vi "Filling.vi"(0 "reference in":refnum<class "Stand.lvclass">, 1 "init":bool, 11 "error in (no error)":errorcluster) -> (4 "reference out":refnum<class "Stand.lvclass">, 15 "error out":errorcluster)   [LabVIEW 2019, in "Stand.lvclass"]
uses:
  Stand.lvclass
  C:/Users/ANENKOV_V1/Desktop/SRC_H400/src/src/Device_class/Device.lvclass
  Device_class/Device.lvclass/Device.ctl
  Stand.lvclass/Stand.ctl
  FPGA/TypeDef/DO index.ctl
  AI_class/AI.lvclass/AI.ctl
  AnalogComparator_class/AnalogComparator.lvclass/AnalogComparator.ctl
  PM_Group_class/PM_Group.lvclass/PM_Group.ctl
  Valve Mode.ctl
  TypeDef/Active Motor.ctl
  TypeDef/Motor N.ctl
  Valve_2DO_2DI_class/CMD.ctl
  TypeDef/Mode.ctl
  AnalogComparator_class/GetStatus.vi
  Valve State Mode.vi
  Valve State Mode.vi/810e184e-eeb6-4027-a8ae-1422f3ce3d45.vi
  Valve State Mode.vi/57bd4a65-f3dc-44f5-8d68-677c2a197570.vi
  Valve State Mode.vi/03b2f9e4-fceb-4725-9b90-3fd10082a088.vi
  Valve State Mode.vi/2785bab5-dd59-4d13-b638-b9157202fa4a.vi
  Valve State Mode.vi/50faa4b8-a9b4-4cc6-ab66-55c42b424fcd.vi
  Valve State Mode.vi/c882c3fe-b7a7-4419-8f9b-6788aa23338b.vi
  Valve State Mode.vi/3d0d09bd-48e8-482f-b1e2-a36b2bb65234.vi
  Valve State Mode.vi/33d3f26a-dc4a-4f56-bf0a-61d04c5d7434.vi
  Valve State Mode.vi/52af9d47-24d1-4057-80bf-8d93bfb3d17d.vi
  Valve State Mode.vi/bbc9916c-129f-4456-975e-9c3ae3d5db66.vi
  Valve State Mode.vi/a6106d78-2bf9-477e-b655-d47fad07ddfe.vi
  Valve State Mode.vi/e2916439-03c6-4471-bb40-42242a636e27.vi
  Valve State Mode.vi/094228cb-a119-423c-9af8-5a16f059a318.vi
  Valve State Mode.vi/bf5ad1e6-a0ae-4579-ad74-ca8f304cb7cf.vi
  Valve State Mode.vi/eb4d2b76-f0f0-4e1d-bda0-609c5f37b4e7.vi
  Const All Valve.vi
  FPGA/TypeDef/AI index.ctl
  FPGA_API_class/FPGA API.lvclass
  AI_class/AI.lvclass
  Device_class/Device.lvclass
  PM_Group_class/PM_Group.lvclass
  Valve_2DO_2DI_class/Valve_2DO_2DI.lvclass
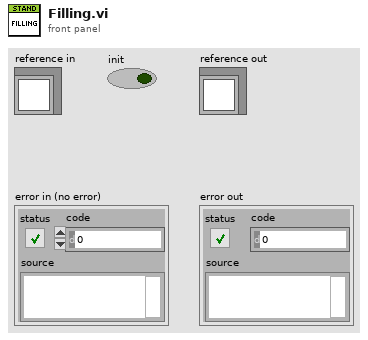
[diagram p1: front panel]
types:
  T1 = typedef "Valve Mode.ctl" = enum16{"Filling DUT", "Filling Chamber", "Pump Pressure DUT", "Pump Pressure Chamber", "Haskel Pressure DUT", "Haskel Pressure Chamber", "Slow Release DUT", "Slow Release Chamber", "Fast Release DUT", "Fast Release Chamber", "Fast Release DUT and Chamber", "Leak Pressure DUT", "Leak Pressure Chamber", "Back Pressure DUT", "Back Pressure Chamber", "Fully Closed", "Drain", "Block DUT", "Block Chamber", "filling dut down", "filling chamber down"}
  T2 = typedef "Active Motor.ctl" = cluster{"Active":bool, "MotorN":T3}
  T3 = typedef "Motor N.ctl" = enum16{"M12", "M21", "M24"}
  T4 = typedef "Valve_2DO_2DI.lvclass/CMD.ctl" = enum16{"Open", "Close"}
  T5 = typedef "DO index.ctl" = u8
  T6 = typedef "AI index.ctl" = u8
  T7 = typedef "Direction.ctl" = enum8{"DUT", "Chamber"}
  T8 = typedef "AI_Data.ctl" = cluster{"Stat Data":T9, "OutOfRangeMax":bool, "OutOfRangeMin":bool, "HIHI":bool, "HI":bool, "LO":bool, "LOLO":bool}
  T9 = typedef "AI Statistics Data.ctl" = cluster{"raw mean":dbl, "scl mean":dbl, "raw mean 1Hz":dbl, "scl mean 1Hz":dbl}
  T10 = typedef "GUI Setting PMG.ctl" = cluster{"Temp Turn ON M24":dbl, "Temp Turn OFF M24":dbl, "Temp Open Water M21":dbl, "Temp Close Water M21":dbl, "delta level":dbl, "fililing level %":dbl, "fililing voltage [V]":dbl}
  T11 = typedef "Mode.ctl" = enum16{"IDLE", "FILLING", "EXECUTE_SP", "DRAIN"}
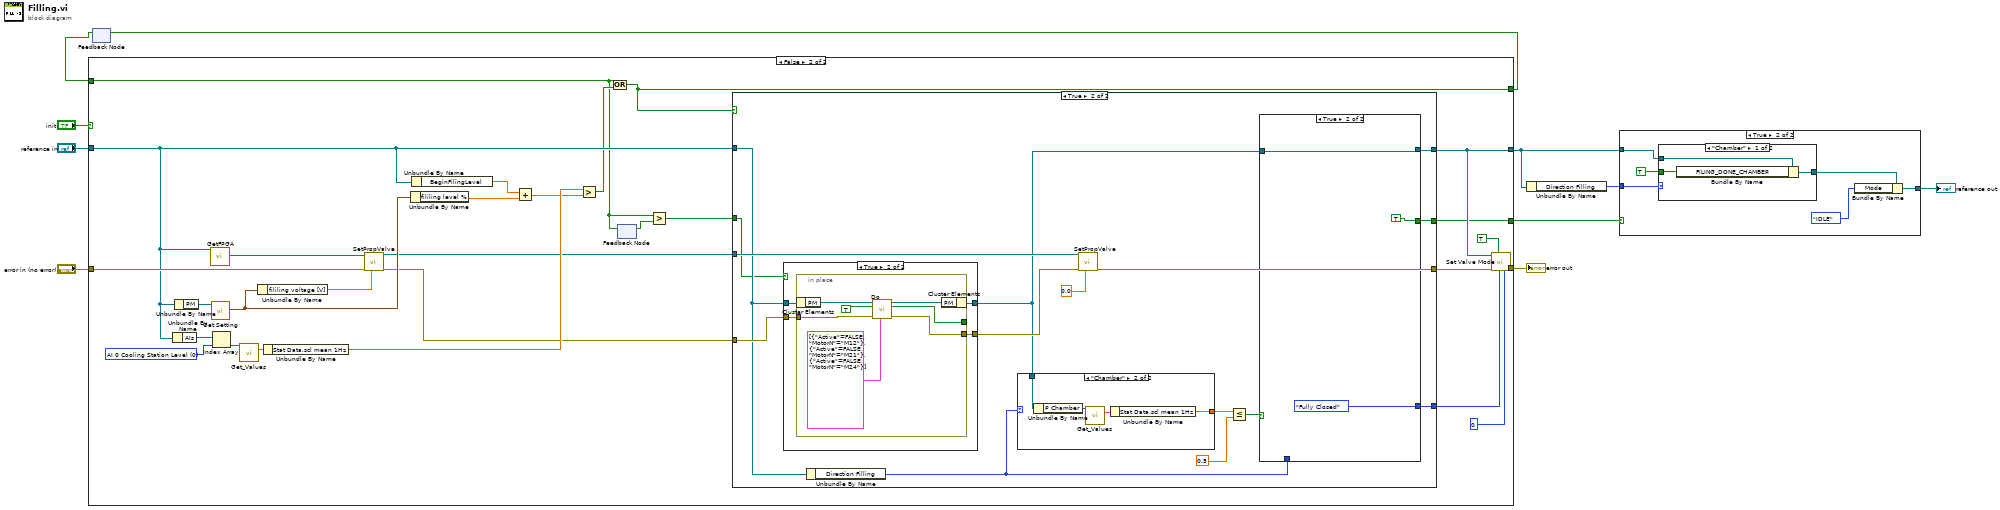
[diagram p0: block diagram]
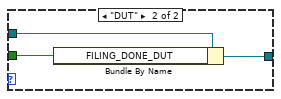
[diagram p3: hidden frame]
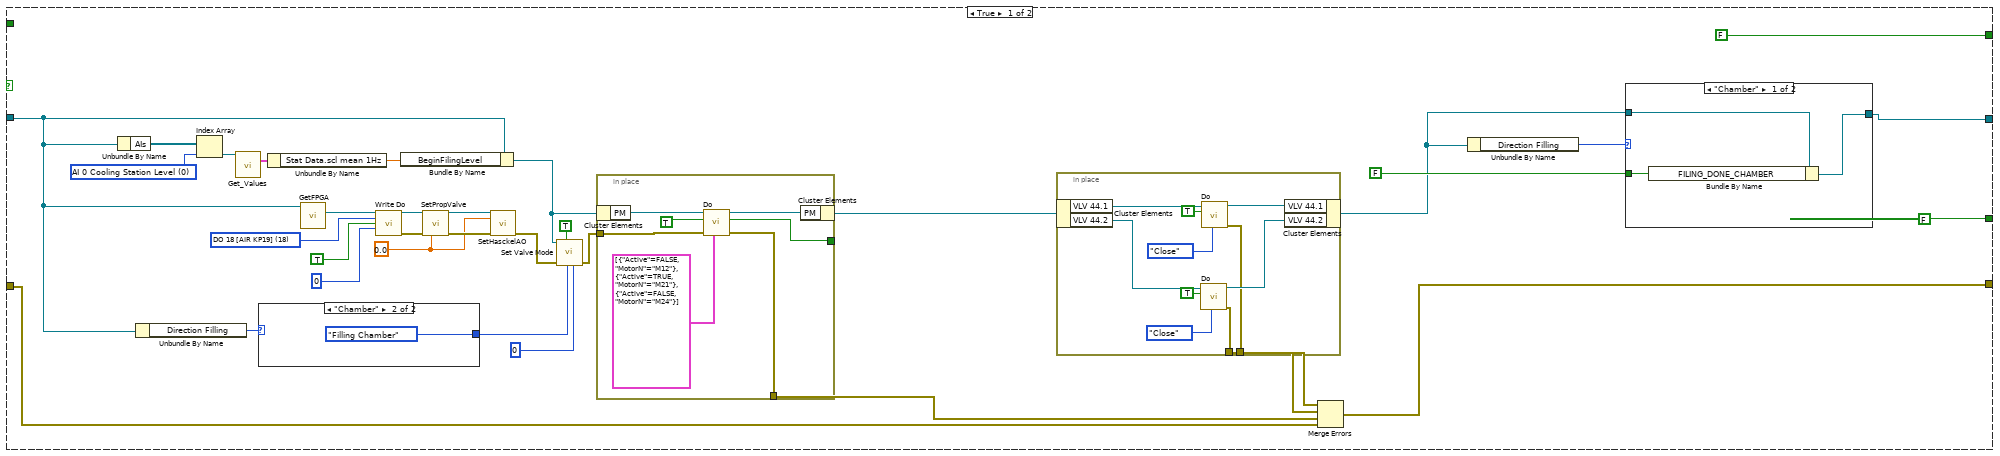
[diagram p4: hidden frame]
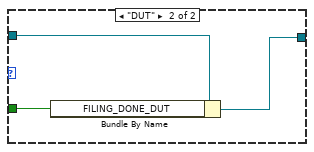
[diagram p5: hidden frame]
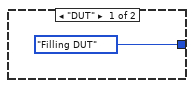
[diagram p6: hidden frame]
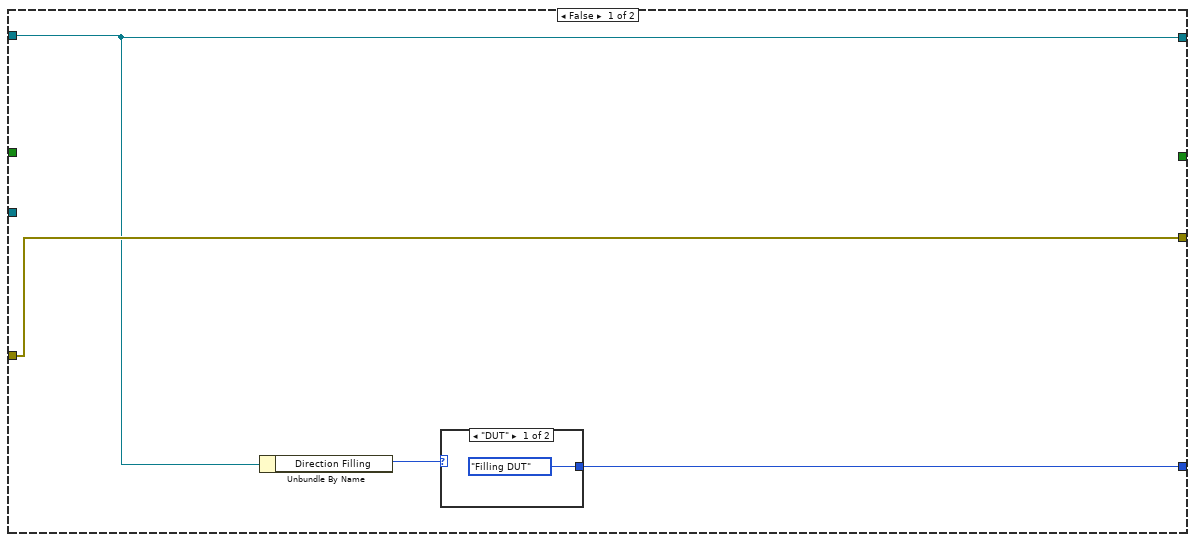
[diagram p7: hidden frame]
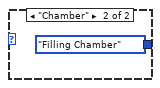
[diagram p8: hidden frame]
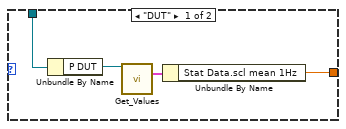
[diagram p10: hidden frame]
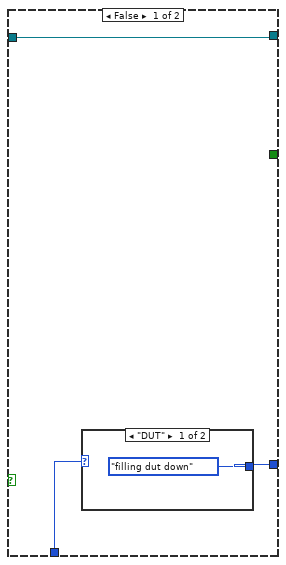
[diagram p11: hidden frame]
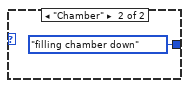
[diagram p12: hidden frame]
diagram:
  n1 = feedback #1() -> (w1:bool)  [unwired: 1 in]
  n2 = case shown="False" "init" {
    tunnel: [w13 w78] -> w4
    tunnel: [w26 w80] -> w10
    tunnel: "error in (no error)" -> [w23 w97]
    tunnel: "reference in" -> [w25 w76]
    tunnel: [FALSE w70] -> w3
    tunnel: [FALSE w74] -> w2
    tunnel: w1 -> [_ w73]
    frame True {
      w30 = 0.0 ("AO 1")
      w29 = T5 18 items=["DO 0 [KP1] [M12]", "DO 1 [ON KP2] [M21]", "DO 2 [ON KP3] [M24]", "DO 3 [WATER Y18.1 [DO3]]", "DO 4 [WATER Y18.2 [DO4]]", "DO 5 [KP6 Y29.1 33.7]", "DO 6 [KP7 Y29.2 33.8]", "DO 7 [KP8 Y29.3 33.9]", "DO 8 [KP9 Y29.4  33.12]", "DO 9 [KP10 Y29.5 33.1]", "DO 10 [KP11 Y29.6 33.2]", "DO 11 [KP12 Y29.7  33.13]", "DO 12 [KP13 Y29.8  33.11]", "DO 13 [KP14 Y29.9 33.10]", "DO 14 [KP15 Y29.10  33.6]", "DO 15 [KP16 Y29.11  33.5]", "DO 16 [KP17 Y29.12  33.4]", "DO 17 [KP18 Y29.13 33.3]", "DO 18 [AIR KP19]", "DO 19 [STEP DRIVE EN KP20]", "DO 20 [KP21 Y44.1 OPEN]", "DO 21 [ KP22 Y44.1 CLOSE]", "DO 22 [ KP23 Y44.2 OPEN]", "DO 23", "DO 24 [STEP DRIVE 1]", "DO 25 [STEP DRIVE 2]"] ("#DO")
      w41 = T6 0 items=["AI 0 Cooling Station Level", "AI 1 Cooling Station Temp", "AI 2 Oil Supply Level", "AI 3 Oil Supply Temp", "AI 4 ", "AI 5 Pressure Haskel", "AI 6 Pressure DUT", "AI 7 Pressure Chamber", "AI 8 Pressure Air inlet", "AI 9 Pressure Air outlet", "AI 10 Pressure Messure Line"] ("AI index")
      n3 = Unbundle By Name(w25) -> ("AIs"=w42:refnum<class "AI.lvclass">[])
      n4 = Unbundle By Name(w25) -> ("Direction Filling"=w24:T7)
      n5 = Index Array(array=w42, index=w41) -> (element=w43:refnum<class "AI.lvclass">)
      n6 = call "Get_Values.vi"("reference in"=w43) -> ("Data"=w40:T8)  [unwired: 14 in]
      n7 = case shown="\"Chamber\"" w24 {
        tunnel: [Valve_Mode."Filling DUT" ("Valve DIR") Valve_Mode."Filling Chamber" ("Valve DIR")] -> w18
        frame "DUT" {
        }
        frame "Chamber" {
        }
      }
      n8 = Unbundle By Name(w40) -> ("Stat Data.scl mean 1Hz"=w44:dbl)
      n9 = call "GetFPGA.vi"("Device in"=w25) -> ("FPGA API.lvclass"=w35:refnum<class "FPGA API.lvclass">)  [unwired: 10 in]
      n10 = call-dynamic "Write Do.vi"("FPGA API in"=w35, "#DO"=w29, "value"=TRUE, "Time uSec"=u32 0) -> ("FPGA API out"=w34:refnum<class "FPGA API.lvclass">, "error out"=w33:errorcluster)  [unwired: 10 in]
      n11 = Bundle By Name(cluster=w25, "BeginFilingLevel"=w44) -> (w20:refnum<class "Stand.lvclass">)
      n12 = call-dynamic "SetPropValve.vi"("FPGA API in"=w34, "error in (no error)"=w33, "AO 1"=w30) -> ("FPGA API out"=w32:refnum<class "FPGA API.lvclass">, "error out"=w31:errorcluster)  [unwired: 11 in]
      n13 = call-dynamic "SetHasckelAO.vi"("FPGA API in"=w32, "Haskel in"=w30, "error in (no error)"=w31) -> ("error out"=w21:errorcluster)  [unwired: 11 in, 1 out]
      n14 = call "Set Valve Mode.vi"("time after close"=u32 0, "Valve DIR"=w18, "init"=TRUE, "error in (no error)"=w21, "Stand in"=w20) -> ("error out"=w22:errorcluster)  [unwired: 5 in, 1 out]
      n15 = in-place {
        in-place-border: w22 -> [w58]
        in-place-border: [w56] -> w36
        in-place-border: [w53] -> _
        n16 = in-place-cluster #2(w20) -> ("PM"=w59:refnum<class "PM_Group.lvclass">)
        n17 = call "Do.vi"("Data"=T2[] [{"Active"=FALSE, "MotorN"=enum."M12"}, {"Active"=TRUE, "MotorN"=enum."M21"}, {"Active"=FALSE, "MotorN"=enum."M24"}] ("Array"), "error in (no error)"=w58, "Do"=TRUE, "PM_Group in"=w59) -> ("error out"=w56:errorcluster, "Done"=w53:bool, "PM_Group out"=w57:refnum<class "PM_Group.lvclass">)  [unwired: 5 in]
        n18 = in-place-cluster #2("PM"=w57) -> (w37:refnum<class "Stand.lvclass">)
      }
      n19 = in-place {
        in-place-border: [w61] -> w39
        in-place-border: [w60] -> w38
        n20 = in-place-cluster #3(w37) -> ("VLV 44.1"=w69:refnum<class "Valve_2DO_2DI.lvclass">, "VLV 44.2"=w63:refnum<class "Valve_2DO_2DI.lvclass">)
        n21 = call "Do.vi"("CMD"=CMD."Close", "Do"=TRUE, "Valve_2DO_2DI in"=w63) -> ("error out"=w61:errorcluster, "Valve_2DO_2DI out"=w62:refnum<class "Valve_2DO_2DI.lvclass">)  [unwired: 6 in, 1 out]
        n22 = call "Do.vi"("CMD"=CMD."Close", "Do"=TRUE, "Valve_2DO_2DI in"=w69) -> ("error out"=w60:errorcluster, "Valve_2DO_2DI out"=w68:refnum<class "Valve_2DO_2DI.lvclass">)  [unwired: 6 in, 1 out]
        n23 = in-place-cluster #3("VLV 44.1"=w68, "VLV 44.2"=w62) -> (w15:refnum<class "Stand.lvclass">)
      }
      n24 = Merge Errors(w38, w39, w36, w23) -> (w26:errorcluster)
      n25 = Unbundle By Name(w15) -> ("Direction Filling"=w14:T7)
      n26 = case shown="\"Chamber\"" w14 {
        tunnel: FALSE -> [w47 w50]
        tunnel: [w46 w49] -> w13
        tunnel: w15 -> [w45 w48]
        frame "Chamber" {
          n27 = Bundle By Name(cluster=w45, "FILING_DONE_CHAMBER"=w47) -> (w46:refnum<class "Stand.lvclass">)
        }
        frame "DUT" {
          n28 = Bundle By Name(cluster=w48, "FILING_DONE_DUT"=w50) -> (w49:refnum<class "Stand.lvclass">)
        }
      }
    }
    frame False {
      w86 = T6 0 items=["AI 0 Cooling Station Level", "AI 1 Cooling Station Temp", "AI 2 Oil Supply Level", "AI 3 Oil Supply Temp", "AI 4 ", "AI 5 Pressure Haskel", "AI 6 Pressure DUT", "AI 7 Pressure Chamber", "AI 8 Pressure Air inlet", "AI 9 Pressure Air outlet", "AI 10 Pressure Messure Line"] ("AI index")
      n29 = Unbundle By Name(w76) -> ("AIs"=w87:refnum<class "AI.lvclass">[])
      n30 = Unbundle By Name(w76) -> ("PM"=w90:refnum<class "PM_Group.lvclass">)
      n31 = call "GetFPGA.vi"("Device in"=w76) -> ("FPGA API.lvclass"=w89:refnum<class "FPGA API.lvclass">)  [unwired: 10 in]
      n32 = call "Get Setting.vi"("PM_Group in"=w90) -> ("Setting PMG"=w92:T10)  [unwired: 9 in, 1 out]
      n33 = Index Array(array=w87, index=w86) -> (element=w88:refnum<class "AI.lvclass">)
      n34 = call "Get_Values.vi"("reference in"=w88) -> ("Data"=w85:T8)  [unwired: 14 in]
      n35 = Unbundle By Name(w92) -> ("fililing voltage [V]"=w93:dbl)
      n36 = Unbundle By Name(w85) -> ("Stat Data.scl mean 1Hz"=w96:dbl)
      n37 = call-dynamic "SetPropValve.vi"("FPGA API in"=w89, "error in (no error)"=w97, "AO 1"=w93) -> ("FPGA API out"=w83:refnum<class "FPGA API.lvclass">, "error out"=w84:errorcluster)  [unwired: 11 in]
      n38 = Unbundle By Name(w92) -> ("fililing level %"=w91:dbl)
      n39 = Unbundle By Name(w76) -> ("BeginFilingLevel"=w94:dbl)
      n40 = Add(x=w94, y=w91) -> (x+y=w95:dbl)
      n41 = Greater?(x=w96, y=w95) -> (0:w75:bool)
      n42 = Or(x=w73, y=w75) -> (x .or. y?=w74:bool)
      n43 = feedback-in #4(w73) -> ()
      n44 = feedback #4() -> (w72:bool)  [unwired: 1 in]
      n45 = Greater?(x=w73, y=w72) -> (0:w71:bool)
      n46 = case shown="True" w74 {
        tunnel: w76 -> [w99 w111]
        tunnel: w84 -> [w101 w118]
        tunnel: w83 -> [_ w117]
        tunnel: [w101 w116] -> w81
        tunnel: [w99 w114] -> w78
        tunnel: [w98 w112] -> w77
        tunnel: w71 -> [_ w105]
        tunnel: [_ w104] -> w70
        frame False {
          n47 = Unbundle By Name(w99) -> ("Direction Filling"=w100:T7)
          n48 = case shown="\"DUT\"" w100 {
            tunnel: [Valve_Mode."Filling DUT" ("Valve DIR") Valve_Mode."Filling Chamber" ("Valve DIR")] -> w98
            frame "DUT" {
            }
            frame "Chamber" {
            }
          }
        }
        frame True {
          n49 = case shown="True" w105 {
            tunnel: w118 -> [w119 w124]
            tunnel: [w119 w123] -> w113
            tunnel: w111 -> [w120 w122]
            tunnel: [w120 w121] -> w109
            frame False {
            }
            frame True {
              n50 = in-place {
                in-place-border: w124 -> [w130]
                in-place-border: [w126] -> _
                in-place-border: [w125] -> w123
                n51 = in-place-cluster #5(w122) -> ("PM"=w131:refnum<class "PM_Group.lvclass">)
                n52 = call "Do.vi"("Data"=T2[] [{"Active"=FALSE, "MotorN"=enum."M12"}, {"Active"=FALSE, "MotorN"=enum."M21"}, {"Active"=FALSE, "MotorN"=enum."M24"}] ("Array"), "error in (no error)"=w130, "Do"=TRUE, "PM_Group in"=w131) -> ("error out"=w125:errorcluster, "Done"=w126:bool, "PM_Group out"=w129:refnum<class "PM_Group.lvclass">)  [unwired: 5 in]
                n53 = in-place-cluster #5("PM"=w129) -> (w121:refnum<class "Stand.lvclass">)
              }
            }
          }
          n54 = Unbundle By Name(w111) -> ("Direction Filling"=w110:T7)
          n55 = case shown="\"Chamber\"" w110 {
            tunnel: w109 -> [w133 w137]
            tunnel: [w132 w136] -> w107
            frame "DUT" {
              n56 = Unbundle By Name(w133) -> ("P DUT"=w134:refnum<class "AI.lvclass">)
              n57 = call "Get_Values.vi"("reference in"=w134) -> ("Data"=w135:T8)  [unwired: 14 in]
              n58 = Unbundle By Name(w135) -> ("Stat Data.scl mean 1Hz"=w132:dbl)
            }
            frame "Chamber" {
              n59 = Unbundle By Name(w137) -> ("P Chamber"=w138:refnum<class "AI.lvclass">)
              n60 = call "Get_Values.vi"("reference in"=w138) -> ("Data"=w139:T8)  [unwired: 14 in]
              n61 = Unbundle By Name(w139) -> ("Stat Data.scl mean 1Hz"=w136:dbl)
            }
          }
          n62 = call-dynamic "SetPropValve.vi"("FPGA API in"=w117, "error in (no error)"=w113, "AO 1"=0.0) -> ("error out"=w116:errorcluster)  [unwired: 11 in, 1 out]
          n63 = Less Or Equal?(x=w107, y=0.5) -> (x <= y?=w108:bool)
          n64 = case shown="True" w108 {
            tunnel: [w141 w147] -> w114
            tunnel: w109 -> [w141 w147]
            tunnel: [w142 Valve_Mode."Fully Closed" ("Valve DIR")] -> w112
            tunnel: w110 -> [w140 _]
            tunnel: [_ TRUE] -> w104
            frame False {
              n65 = case shown="\"DUT\"" w140 {
                tunnel: [Valve_Mode."filling dut down" ("Valve DIR") Valve_Mode."filling chamber down" ("Valve DIR")] -> w142
                frame "DUT" {
                }
                frame "Chamber" {
                }
              }
            }
            frame True {
            }
          }
        }
      }
      n66 = call "Set Valve Mode.vi"("time after close"=u32 0, "Valve DIR"=w77, "init"=TRUE, "error in (no error)"=w81, "Stand in"=w78) -> ("error out"=w80:errorcluster)  [unwired: 5 in, 1 out]
    }
  }
  "error out" <- w10
  n67 = feedback-in #1(w2) -> ()
  n68 = Unbundle By Name(w4) -> ("Direction Filling"=w6:T7)
  n69 = case shown="True" w3 {
    tunnel: w6 -> [_ w154]
    tunnel: [w148 w149] -> w5
    tunnel: w4 -> [w148 w152]
    frame False {
    }
    frame True {
      n70 = case shown="\"Chamber\"" w154 {
        tunnel: TRUE -> [w157 w160]
        tunnel: [w156 w159] -> w150
        tunnel: w152 -> [w155 w158]
        frame "Chamber" {
          n71 = Bundle By Name(cluster=w155, "FILING_DONE_CHAMBER"=w157) -> (w156:refnum<class "Stand.lvclass">)
        }
        frame "DUT" {
          n72 = Bundle By Name(cluster=w158, "FILING_DONE_DUT"=w160) -> (w159:refnum<class "Stand.lvclass">)
        }
      }
      n73 = Bundle By Name(cluster=w150, "Mode"=Mode."IDLE" ("Data.Mode")) -> (w149:refnum<class "Stand.lvclass">)
    }
  }
  "reference out" <- w5
